vi "toDevULong.vi"(1 "ArgIO":cluster{"num data":u8[], "str data":string[]}) -> (0 "argout":u32)   [LabVIEW 2014, in "tango.lvlib"]
uses:
  tango.lvlib
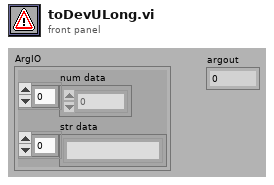
[diagram p1: front panel]
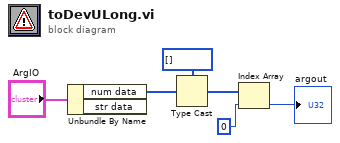
[diagram p0: block diagram]
diagram:
  n1 = Unbundle By Name("ArgIO") -> ("num data"=w1:u8[])  [unwired: 1 out]
  n2 = Type Cast(type=u32[] [], x=w1) -> (*(type *) &x=w2:u32[])
  n3 = Index Array(array=w2, index=0 ("indice")) -> (element=→"argout":u32)
